vi "Counter - Read Pulse Width and Frequency (Finite).vi"() -> ()   [LabVIEW 2022 SP3]
doc: "This example demonstrates how to measure a finite number of samples of period, frequency, pulse width, or two edge separation measurements.\n\nThis example uses implicit timing, which means that a sample is acquired for every period of your input signal.\n\nFor instructions on how to connect your signals to the DAQ device, refer to your device documentation."
uses:
  <vilib>/Utility/error.llb/DialogType.ctl
  <vilib>/DAQmx/read.llb/DAQmx Read (Counter 1D DBL 1Chan NSamp).vi
  <vilib>/DAQmx/create/channels.llb/DAQmx Create Channel (CI-Period).vi
  <vilib>/DAQmx/create/channels.llb/DAQmx Create Channel (CI-Frequency).vi
  <vilib>/DAQmx/create/channels.llb/DAQmx Create Channel (CI-Pulse Width).vi
  <vilib>/DAQmx/create/channels.llb/DAQmx Create Channel (CI-Two Edge Separation).vi
  <vilib>/DAQmx/configure/timing.llb/DAQmx Timing (Implicit).vi
  <vilib>/DAQmx/miscellaneous.llb/DAQmx Fill In Error Info.vi
  <resource>/objmgr/daqmx.rc
panel:
  out "Data":dbl[](array[numeric])
  in  "Counter Input Type":T1(tab)
  in  "Period Input Terminal":tag="/Dev1/PFI9"
  in  "Max Period":dbl=0.1 format="%0.6f"
  in  "Min Period":dbl=1e-06 format="%0.6f"
  in  "Min Frequency":dbl=2.0 format="%0.6f"
  in  "Max Frequency":dbl=100.0 format="%0.6f"
  in  "Frequency Input Terminal":tag="/Dev1/PFI9"
  in  "Pulse Width Input Terminal":tag="/Dev1/PFI9"
  in  "Min Pulse Width":dbl=1e-06 format="%0.6f"
  in  "Max Pulse Width":dbl=0.1 format="%0.6f"
  in  "Second Input Terminal":tag="/Dev1/PFI9"
  in  "Frst Input Terminal":tag="/Dev1/PFI10"
  in  "Min Separation Time":dbl=1e-06 format="%0.6f"
  in  "Max Separation Time":dbl=0.1 format="%0.6f"
  in  "Number of Samples":i32=1000
  in  "Counter":tag="Dev1/ctr0"
  # "Channel Settings"
  # "Acquired Data"
  # "Timing Settings"
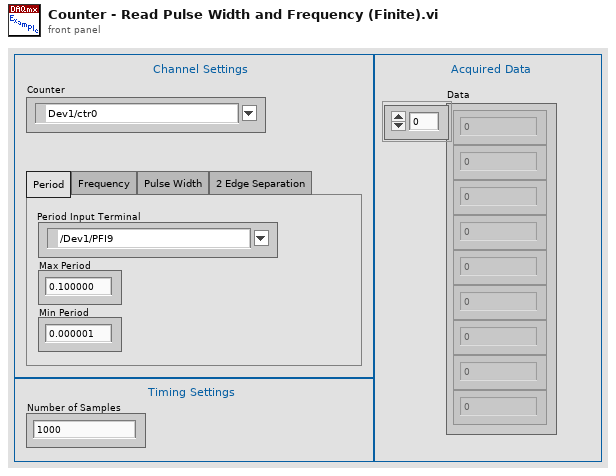
[diagram p1: front panel]
types:
  T1 = enum32{"Period", "Frequency", "Pulse Width", "2 Edge Separation"}
  T2 = typedef "DialogType.ctl" = u16
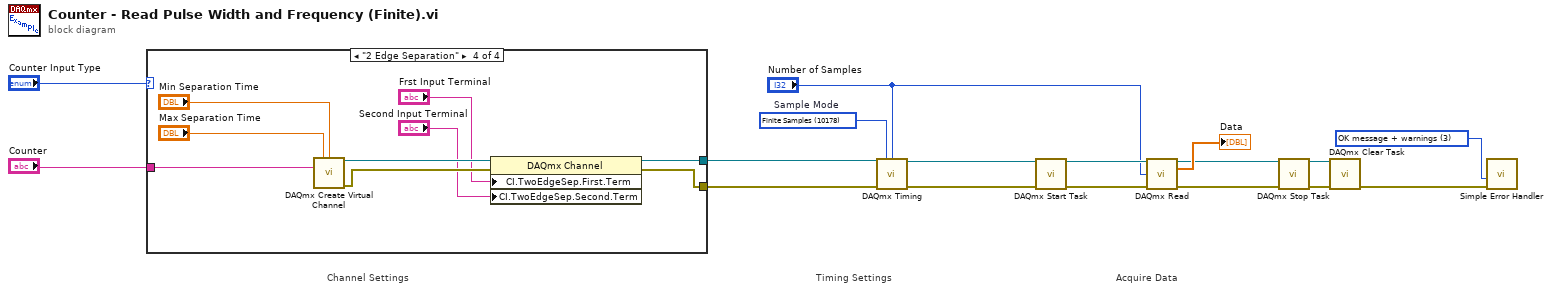
[diagram p0: block diagram]
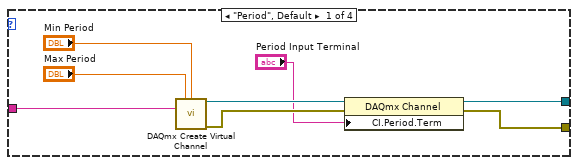
[diagram p2: hidden frame]
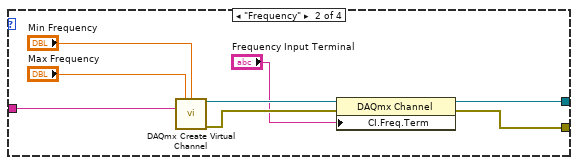
[diagram p3: hidden frame]
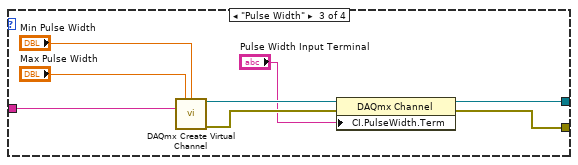
[diagram p4: hidden frame]
diagram:
  w1 = T2 3 items=["no dialog", "OK message", "continue or stop message", "OK message + warnings", "continue/stop + warnings"] ("type of dialog (OK msg:1)")
  w17 = 10178 items=["Finite Samples"=10178, "Continuous Samples"=10123, "Hardware Timed Single Point"=12522]  # Sample Mode
  # "Acquire Data"
  # "Timing Settings"
  # "Channel Settings"
  n1 = case shown="\"2 Edge Separation\"" "Counter Input Type" {
    tunnel: [w23 w31 w39 w48] -> w16
    tunnel: [w24 w32 w40 w49] -> w15
    tunnel: "Counter" -> [w25 w33 w41 w50]
    frame "Period", Default {
      n2 = call-poly <vilib>:"DAQmx Create Virtual Channel.vi"("maximum value"="Max Period", "minimum value"="Min Period", "counter"=w25) -> ("task out"=w22:refnum<k21>, "error out"=w21:errorcluster)  [unwired: 11 in]
      n3 = property class="DAQmx Channel"(reference=w22, error in=w21, "CI.Period.Term"="Period Input Terminal") -> (reference out=w24:refnum<k21>, error out=w23:errorcluster)
    }
    frame "Frequency" {
      n4 = call-poly <vilib>:"DAQmx Create Virtual Channel.vi"("maximum value"="Max Frequency", "minimum value"="Min Frequency", "counter"=w33) -> ("task out"=w30:refnum<k21>, "error out"=w29:errorcluster)  [unwired: 11 in]
      n5 = property class="DAQmx Channel"(reference=w30, error in=w29, "CI.Freq.Term"="Frequency Input Terminal") -> (reference out=w32:refnum<k21>, error out=w31:errorcluster)
    }
    frame "Pulse Width" {
      n6 = call-poly <vilib>:"DAQmx Create Virtual Channel.vi"("maximum value"="Max Pulse Width", "minimum value"="Min Pulse Width", "counter"=w41) -> ("task out"=w38:refnum<k21>, "error out"=w37:errorcluster)  [unwired: 11 in]
      n7 = property class="DAQmx Channel"(reference=w38, error in=w37, "CI.PulseWidth.Term"="Pulse Width Input Terminal") -> (reference out=w40:refnum<k21>, error out=w39:errorcluster)
    }
    frame "2 Edge Separation" {
      n8 = call-poly <vilib>:"DAQmx Create Virtual Channel.vi"("maximum value"="Max Separation Time", "minimum value"="Min Separation Time", "counter"=w50) -> ("task out"=w47:refnum<k21>, "error out"=w46:errorcluster)  [unwired: 11 in]
      n9 = property class="DAQmx Channel"(reference=w47, error in=w46, "CI.TwoEdgeSep.First.Term"="Frst Input Terminal", "CI.TwoEdgeSep.Second.Term"="Second Input Terminal") -> (reference out=w49:refnum<k21>, error out=w48:errorcluster)
    }
  }
  n10 = call-poly <vilib>:"DAQmx Timing.vi"("task/channels in"=w15, "sample mode"=w17, "samples per channel"="Number of Samples", "error in"=w16) -> ("task out"=w9:refnum<k21>, "error out"=w8:errorcluster)  [unwired: 10 in]
  n11 = call <vilib>:"DAQmx Start Task.vi"("task/channels in"=w9, "error in"=w8) -> ("task out"=w14:refnum<k21>, "error out"=w13:errorcluster)  [unwired: 12 in]
  n12 = call-poly <vilib>:"DAQmx Read.vi"("task/channels in"=w14, "number of samples per channel"="Number of Samples", "error in"=w13) -> ("task out"=w3:refnum<k21>, "data"=→"Data":dbl[], "error out"=w2:errorcluster)  [unwired: 10 in]
  n13 = call <vilib>:"DAQmx Stop Task.vi"("task/channels in"=w3, "error in"=w2) -> ("task out"=w5:refnum<k21>, "error out"=w4:errorcluster)  [unwired: 12 in]
  n14 = call <vilib>:"DAQmx Clear Task.vi"("task in"=w5, "error in"=w4) -> ("error out"=w12:errorcluster)  [unwired: 13 in]
  n15 = call <vilib>:"Simple Error Handler.vi"("type of dialog (OK msg:1)"=w1, "error in (no error)"=w12) -> ()  [unwired: 3 in, 5 out]
